vi "Chain2.vi"(7 "Name (\"\" to Use UUID)":string="CSM-Module") -> ()   [LabVIEW 2017, in "CSM-Testcase.lvlib"]
doc: "Creates a template for a CSM module without a user interface.\n\n> [!NOTE] CSM Name Rules\n> - The CSM module name must be unique to avoid entering the \"Critical Error\" state.\n> - If the input is \"\", a UUID will be used as the module name. This module will operate in independent mode and will not be listed in the module list.\n> - If the input ends with '#', the module will run in work mode. Modules with the same name will share the same message queue. External messages will be handled by the idle module.\n\n> [!NOTE] CSM Initialization State\n> - The default value is \"Macro: Initialize\", consistent with the JKISM state machine.\n> - This state is typically not modified and is provided to facilitate external programmatic changes to the initialization state.\n\n\n-- <b>Controls</b> --\n- <b>Name (\"\" to Use UUID)</b>: CSM Module Name\n- <b>Init State(\"Macro: Initialize\")</b>: Initialization State, default is \"Macro: Initialize\""
uses:
  CSM-Testcase.lvlib
  src/user.lib/_NEVSTOP/Communicable State Machine(CSM)/AdvanceAPI/CSM - Revert Arguments-Safe String.vi
  src/user.lib/_NEVSTOP/Communicable State Machine(CSM)/AdvanceAPI/CSM - Make String Arguments Safe.vi
  src/user.lib/_NEVSTOP/Communicable State Machine(CSM)/AdvanceAPI/CSM - Break Down Multiple States String.vi
  src/user.lib/_NEVSTOP/Communicable State Machine(CSM)/AdvanceAPI/CSM - Keywords.vi
  src/user.lib/_NEVSTOP/Communicable State Machine(CSM)/_Shared/Trim Single-line Text.vi
  src/user.lib/_NEVSTOP/Communicable State Machine(CSM)/_Polymophic/Build No-Reply Asynchronous Message with Arguments.vi
  src/user.lib/_NEVSTOP/Communicable State Machine(CSM)/_Polymophic/Build Asynchronous Message with Arguments.vi
  src/user.lib/_NEVSTOP/Communicable State Machine(CSM)/_Polymophic/Build Register Message.vi
  src/user.lib/_NEVSTOP/Communicable State Machine(CSM)/_Polymophic/Build Interrupt Broadcast Message.vi
  src/user.lib/_NEVSTOP/Communicable State Machine(CSM)/Communicable State Machine.lvlib
  src/user.lib/_NEVSTOP/Communicable State Machine(CSM)/addons/Loop-Support/CSM Loop Support.lvlib
panel:
  out "Error Occurred":errorcluster
  out "State History":string
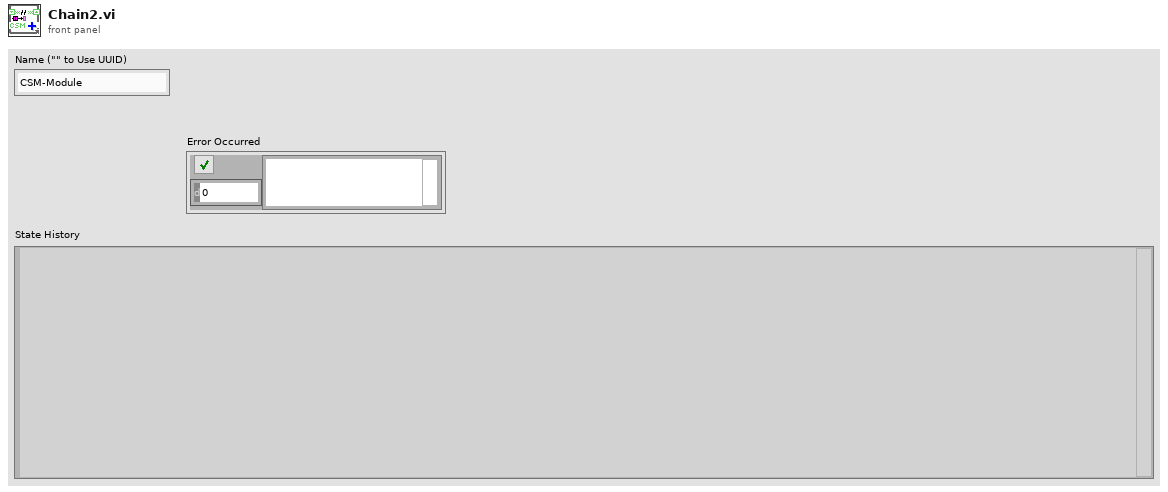
[diagram p1: front panel]
types:
  T1 = cluster{"Arguments":string, "Response":string, "error":errorcluster}
  T2 = enum32{"Invalid", "Standard", "Closed", "Hidden", "Minimized", "Maximized"}
  T3 = enum32{"invalid app kind", "Development System", "Run Time System", "Student Edition", "Embedded LabVIEW", "Evaluation", "Custom"}
  T4 = typedef "Communicable State Machine.lvlib/_CSM_Response Source Message.ctl" = cluster{"‘State":string, "’Arguments":string, "’Error":errorcluster}
  T5 = cluster{"Current VI Reference":refnum<vi>, "Close Panel on Exit?":bool}
  T6 = cluster{"Core":cluster{"Current VI Reference":refnum<vi>, "Close Panel on Exit?":bool}, "Your Boolean data":bool, "Your string data":string, "Counter":u32, "CSM Loop Counter":i32}
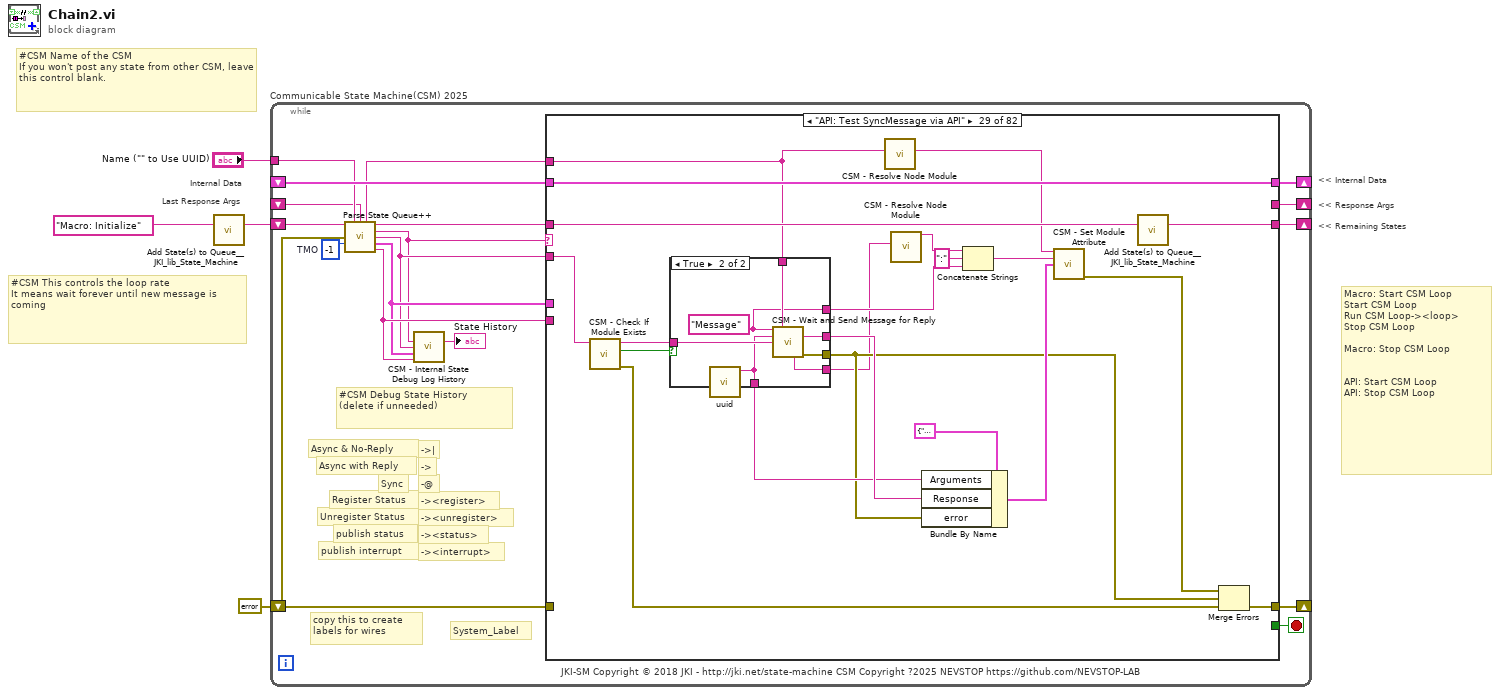
[diagram p0: block diagram]
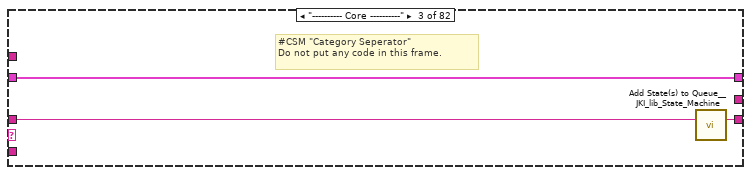
[diagram p4: hidden frame]
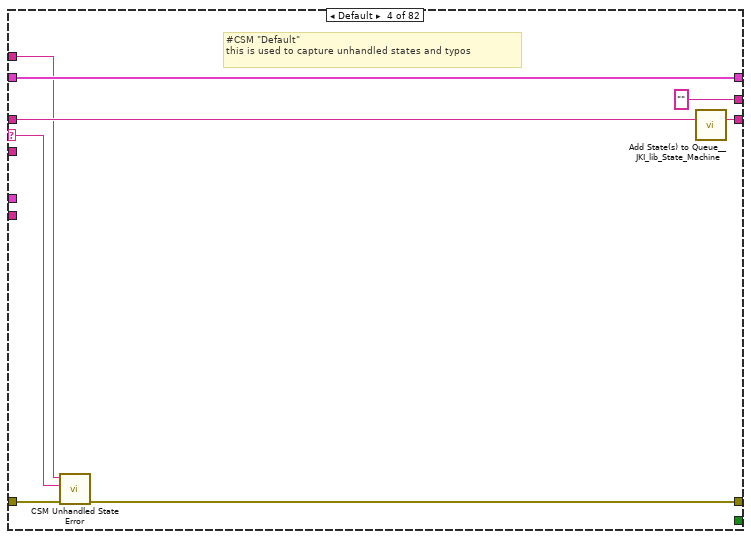
[diagram p5: hidden frame]
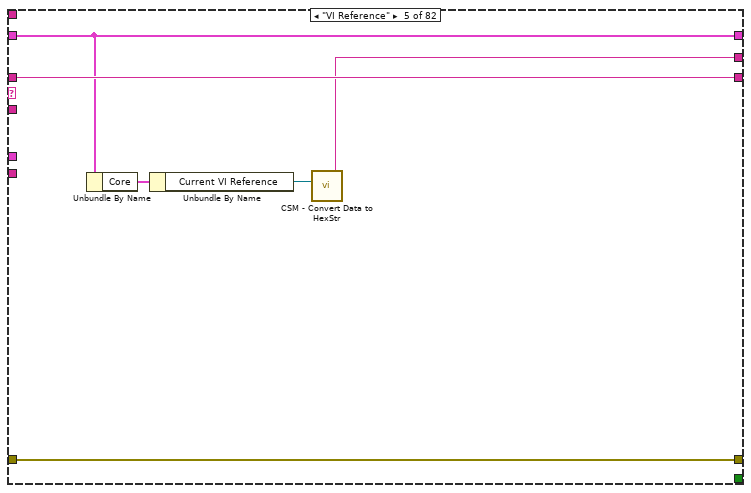
[diagram p6: hidden frame]
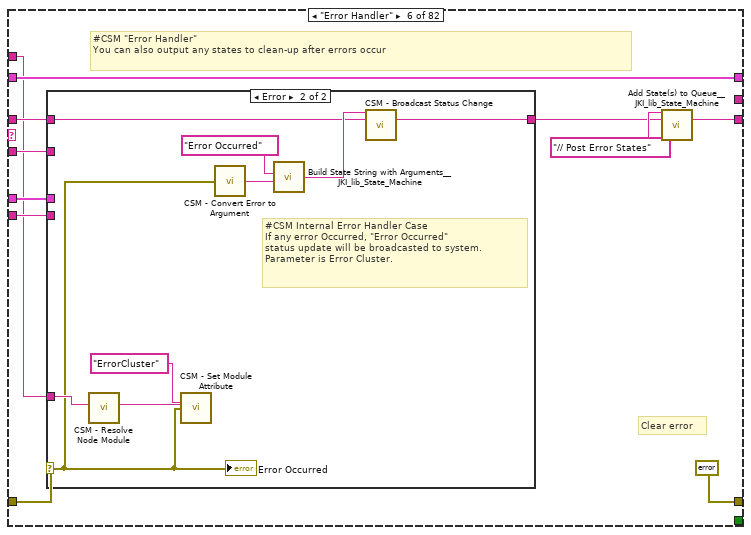
[diagram p7: hidden frame]
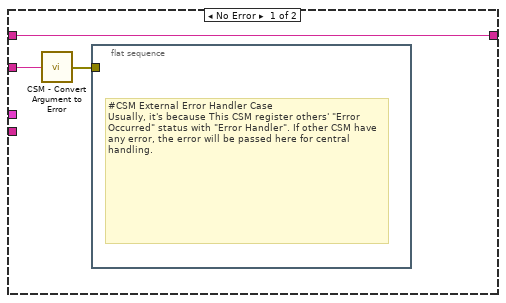
[diagram p8: hidden frame]
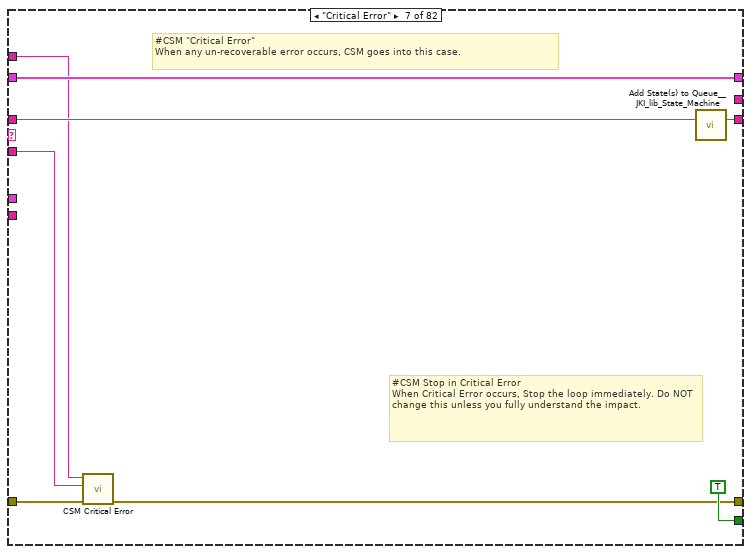
[diagram p9: hidden frame]
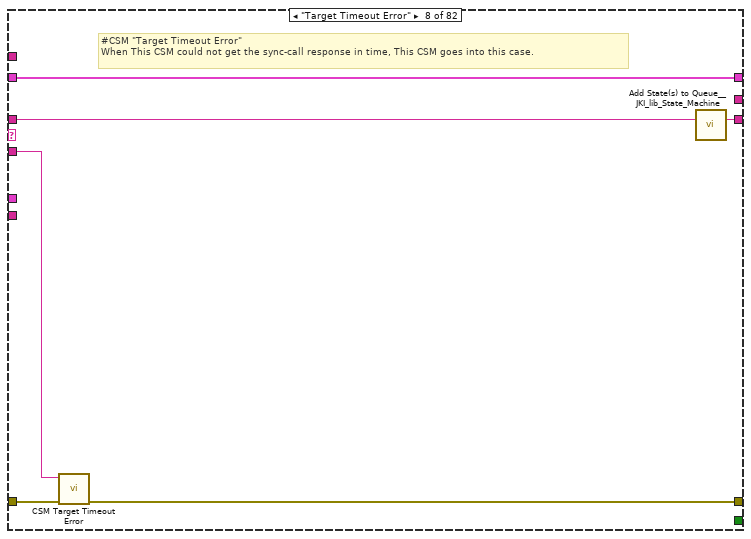
[diagram p10: hidden frame]
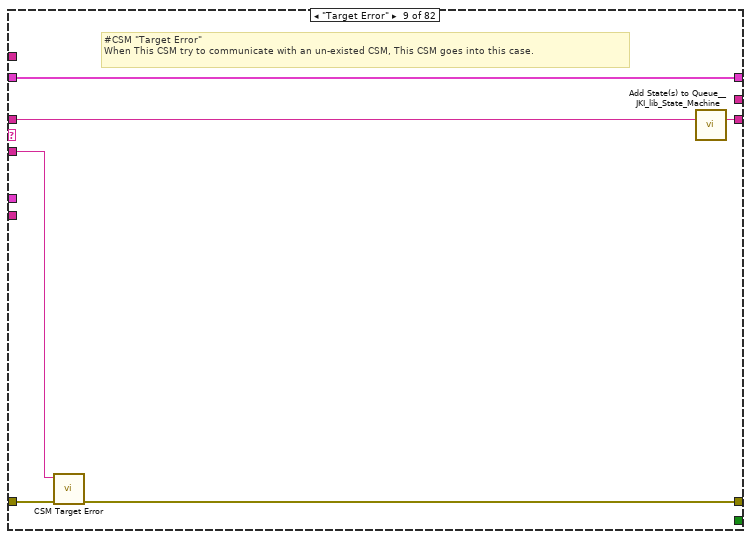
[diagram p11: hidden frame]
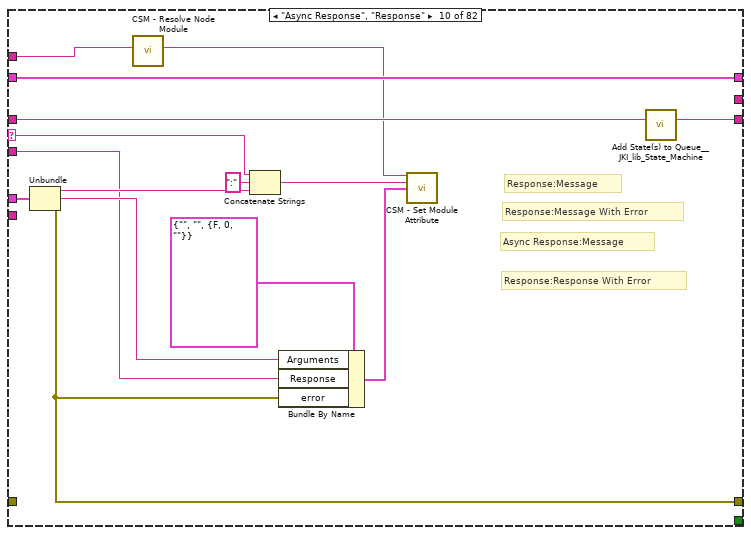
[diagram p12: hidden frame]
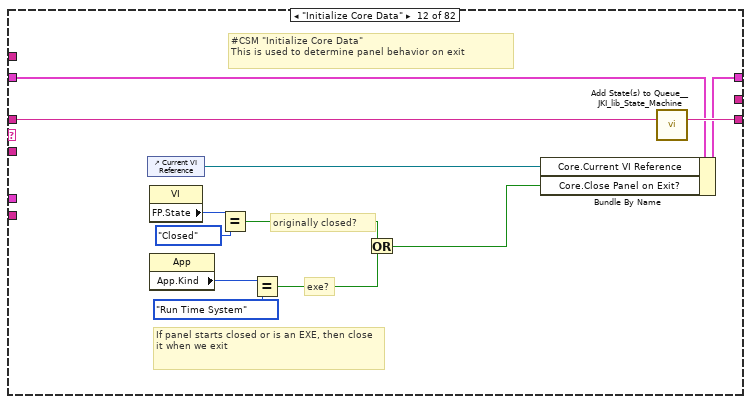
[diagram p14: hidden frame]
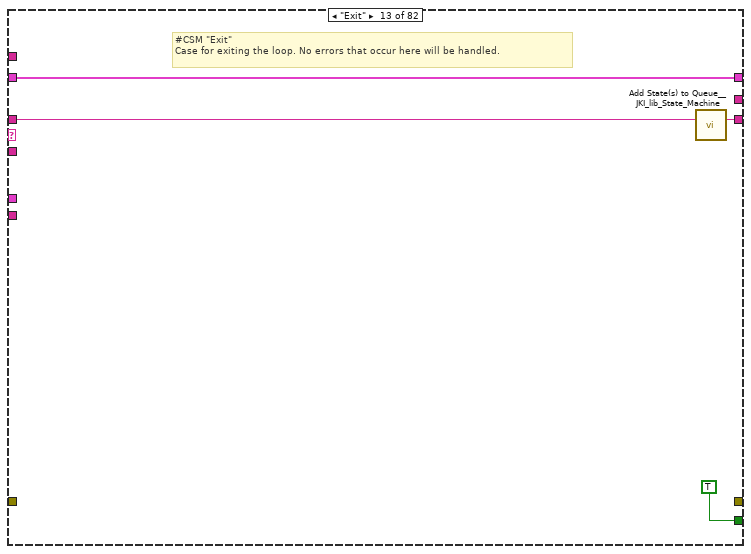
[diagram p15: hidden frame]
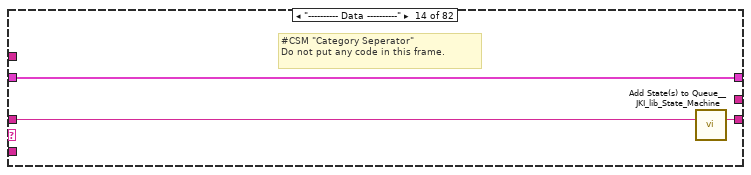
[diagram p16: hidden frame]
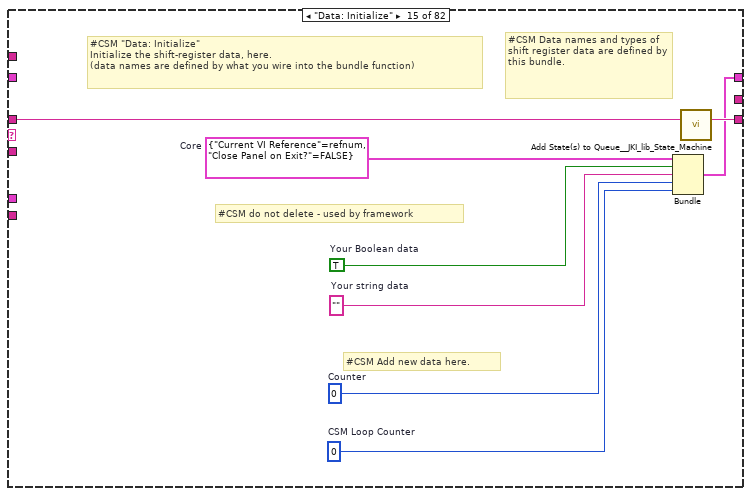
[diagram p17: hidden frame]
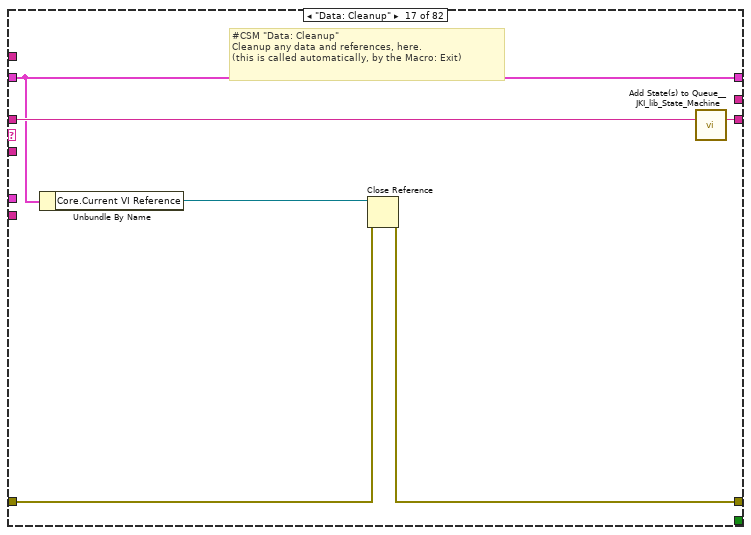
[diagram p19: hidden frame]
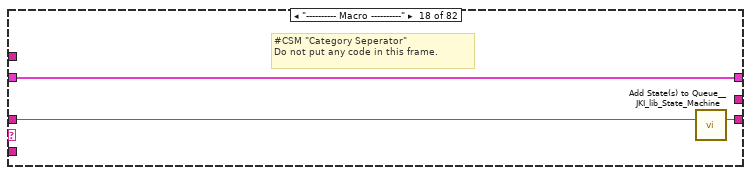
[diagram p20: hidden frame]
diagram:
  # "Macro: Start CSM Loop\nStart CSM Loop\nRun CSM Loop-><loop>\nStop CSM Loop\n\nMacro: Stop CSM Loop\n\n\nAPI: Start CSM Loop\nAPI: Stop CSM Loop"
  # "Last Response Args"
  # "Internal Data"
  # "#CSM Name of the CSM\nIf you won't post any state from other CSM, leave this control blank."
  # "#CSM This controls the loop rate\nIt means wait forever until new message is coming"
  # "<< Internal Data"
  # "<< Response Args"
  # "<< Remaining States"
  n1 = call <vilib>:"Add State(s) to Queue__JKI_lib_State_Machine.vi"("State(s) in (\"\")"="Macro: Initialize" ("Init State(\"Macro: Initialize\")")) -> ("States Out"=w4:string)  [unwired: 14 in]
  n2 = while "Communicable State Machine(CSM) 2025" {
    shift-right: [w17] -> _
    shift-left: _ -> [w16]
    shift-right: [w20] -> _
    shift-left: errorcluster {"status"=FALSE, "code"=0, "source"=""} ("error out") -> [w6]
    shift-right: [w19] -> _
    shift-left: w4 -> [w21]
    tunnel: "Name (\"\" to Use UUID)" -> [w13]
    shift-right: [w14] -> _
    shift-left: _ -> [w8]
    stop <- w18 stop-if-true
    w15 = -1  # TMO
    # "#CSM Debug State History\n(delete if unneeded)"
    # "-><interrupt>"
    # "-><status>"
    # "-><unregister>"
    # "-><register>"
    # "-@"
    # "->"
    # "->|"
    # "publish interrupt"
    # "publish status"
    # "Unregister Status"
    # "Register Status"
    # "Sync"
    # "Async with Reply"
    # "Async & No-Reply"
    # "JKI-SM Copyright © 2018 JKI - http://jki.net/state-machine CSM Copyright ?2025 NEVSTOP https://github.com/NEVSTOP-LAB"
    # "copy this to create labels for wires"
    # "System_Label"
    n3 = call "Parse State Queue++.vi"("State Queue"=w21, "Name (\"\" to Use UUID)"=w13, "Response Arguments"=w8, "Previous Error"=w6, "Dequeue (1 ms)"=w15) -> ("Name Used"=w7:string, "Remaining States"=w22:string, "Current State"=w9:string, "Arguments"=w10:string, "Additional Information"=w11:T4, "Source CSM"=w12:string)  [unwired: 5 in]
    n4 = call "CSM - Internal State Debug Log History.vi"("State"=w9, "Arguments (\"\")"=w10, ">> Response Source Message >>"=w11, "Source (\"\")"=w12) -> ("Debug Log"=→"State History":string)  [unwired: 11 in]
    n5 = case shown="\"API: Test SyncMessage via API\"" w9 {
      selector: w9 -> [_ _ _ w33 _ _ _ _ _ w97 _ _ _ _ _ _ _ _ _ _ _ _ _ _ _ _ _ _ _ _ _ _ _ _ _ _ _ _ _ _ _ _ _ _ _ _ _ _ _ _ _ _ _ _ _ _ _ _ _ w549 w559 _ w573 _ _ _ _ _ _ _ _ _ _ w639 _ _ _ w663 w674 w681 w696 _]
      tunnel: w22 -> [w23 w26 w29 w37 w42 w48 w74 w80 w86 w101 w103 w115 w119 w122 w130 w132 w138 w141 w145 w151 w155 w160 w174 w194 w223 w227 w231 w243 w268 w296 w311 w323 w335 w349 w372 w383 w396 w403 w410 w417 w424 w431 w438 w445 w452 w459 w466 w473 w484 w492 w501 w510 w519 w522 w526 w533 w538 w541 w545 w557 w567 w572 w578 w585 w588 w600 w606 w612 w616 w621 w625 w629 w633 w642 w646 w654 w660 w667 w676 w685 w700 w710]
      tunnel: w10 -> [_ _ _ _ _ w47 w70 w77 w83 w91 _ _ _ _ _ _ _ _ _ _ _ _ w161 w181 w206 _ w234 w246 w271 w299 w314 w326 w338 w352 w368 w386 w393 w400 w407 w414 w421 w428 w435 w442 w449 w456 w463 w470 w477 _ w494 w502 w511 _ _ w531 _ _ _ _ _ w569 _ w581 w590 _ w602 w608 w614 w619 w624 w628 w632 w638 w645 w652 w658 w664 w675 w680 w691 _]
      tunnel: w16 -> [w24 w25 w27 w35 w41 w53 w72 w78 w84 w99 w102 w109 w117 w120 _ w131 w133 w139 w143 w149 w156 w158 w176 w196 w225 w226 w235 w247 w272 w300 w315 w327 w339 w353 w375 w387 w398 w405 w412 w419 w426 w433 w440 w447 w454 w461 w468 w475 w482 w490 w499 w508 w517 w523 w528 w532 w536 w539 w544 w555 w565 w570 w579 w586 w592 w601 w607 w613 w618 w623 w626 w630 w634 w643 w647 w653 w659 w668 w677 w686 w693 w708]
      tunnel: [_ _ _ w30 w43 errorcluster {"status"=FALSE, "code"=0, "source"=""} ("error out") w67 w75 w81 w90 _ _ _ _ _ _ w134 _ _ _ _ _ _ _ _ _ w228 w240 w265 w293 w308 w320 w332 w345 w369 w380 w397 w404 w411 w418 w425 w432 w439 w446 w453 w460 w467 w474 _ _ _ w506 w515 w524 w529 _ _ _ w546 w547 w562 _ _ _ _ _ _ _ w617 w622 w627 w631 w635 w637 w648 w649 w655 w662 w671 w682 w697 _] -> w20
      tunnel: w6 -> [_ _ _ w31 w43 w51 w68 w76 w82 _ _ _ _ _ _ _ w135 _ _ _ _ _ _ _ _ _ _ _ _ _ _ _ _ _ _ _ w397 w404 w411 w418 w425 w432 w439 w446 w453 w460 w467 w474 _ _ _ _ _ w524 w529 _ _ _ w546 _ _ _ _ _ _ _ _ _ w617 w622 w627 w631 w635 w644 w648 w650 w656 w669 w678 w687 w701 _]
      tunnel: [w23 w26 w28 w36 w42 w49 w73 w79 w85 w100 w103 w114 w118 w121 w129 w132 w137 w140 w144 w150 w152 w159 w175 w195 w224 w227 w232 w244 w269 w297 w312 w324 w336 w350 w373 w384 w395 w402 w409 w416 w423 w430 w437 w444 w451 w458 w465 w472 w483 w491 w500 w509 w518 w521 w525 w533 w537 w540 w545 w558 w568 w571 w580 w582 w587 w598 w603 w609 w615 w620 w625 w629 w633 w642 w646 w654 w660 w667 w676 w685 w700 w709] -> w19
      tunnel: [_ _ _ _ _ _ TRUE _ _ _ _ _ TRUE _ _ _ _ _ _ _ _ _ _ _ _ _ _ _ _ _ _ _ _ _ _ _ _ _ _ _ _ _ _ _ _ _ _ _ _ _ _ _ _ _ _ _ _ _ _ _ _ _ _ _ _ _ _ _ _ _ _ _ _ _ _ _ _ _ _ _ _ _] -> w18
      tunnel: [w24 w25 w27 w35 w41 w53 w72 w78 w84 w99 w102 w113 w117 w120 w128 w131 w133 w139 w143 w149 w156 w158 w176 w196 w225 w226 w235 w247 w272 w300 w315 w327 w339 w353 w375 w387 w398 w405 w412 w419 w426 w433 w440 w447 w454 w461 w468 w475 w482 w490 w499 w508 w517 w523 w528 w532 w536 w539 w543 w553 w564 w570 w579 w586 w592 w601 w607 w613 w618 w623 w626 w630 w634 w643 w647 w653 w659 w668 w677 w686 w692 w706] -> w17
      tunnel: w12 -> [_ _ _ _ _ w46 _ _ _ _ _ _ _ _ _ _ _ _ _ _ _ _ _ _ _ _ _ _ _ _ _ _ _ _ _ _ _ _ _ _ _ _ _ _ _ _ _ _ _ _ _ _ _ _ _ _ _ _ _ _ _ _ _ _ _ _ _ _ _ _ _ _ _ _ _ _ _ _ _ _ _ _]
      tunnel: w11 -> [_ _ _ _ _ w45 _ _ _ w98 _ _ _ _ _ _ _ _ _ _ _ _ _ _ _ _ _ _ _ _ _ _ _ _ _ _ _ _ _ _ _ _ _ _ _ _ _ _ _ _ _ _ _ _ _ _ _ _ _ _ _ _ _ _ _ _ _ _ _ _ _ _ _ _ _ _ _ _ _ _ _ _]
      tunnel: [_ _ _ "" w38 _ _ _ _ _ _ _ _ _ _ _ _ _ _ _ _ _ _ _ _ _ _ _ _ _ _ _ _ _ _ _ _ _ _ _ _ _ _ _ _ _ _ _ _ _ _ _ _ _ _ w530 _ _ _ _ _ w569 w574 _ _ _ _ _ w614 w619 w624 w628 w632 w638 w645 w652 w658 _ w675 w680 _ _] -> w14
      tunnel: w7 -> [_ _ _ w32 _ w44 w69 _ _ w88 _ _ _ _ _ _ _ _ _ _ _ _ _ _ _ _ _ _ w256 w284 _ _ _ w346 _ _ _ _ _ _ _ _ _ _ _ _ _ _ w480 w488 w497 w507 w516 _ _ _ _ _ _ w551 w561 _ w575 _ _ w595 _ _ _ _ _ _ _ w641 _ _ _ w666 w673 w684 w699 _]
      frame "", "Idle" {
        # "#CSM \"Idle/Event Handler\"\nexecutes when the state queue is empty"
      }
      frame "CSM Documentation" {
        # "#CSM State Syntax\n\n// Comment line, all text to the right of “//” will be ignored\n// Local Message Example\nDoSth: DoA >> Arguments\n\n// Sync Call Example\nAPI: xxxx >> Arguments -@ TargetModule\n\n// Async Call Example\nAPI: xxxx >> Arguments -> TargetModule\n\n// Async Call without Reply Example\nAPI: xxxx >> Arguments ->| TargetModule\n\n// Broadcast normal status:\nStatus >> StatusArguments  -><status>\n\n// Broadcast Interrupt status:\nInterrupt >> StatusArguments  -><interrupt>\n\n// Register Source Module's status to Handler Module\nStatus@Source Module >> Handler Module@Handler Module -><register>\n\n// Unegister Source Module's status\nStatus@Source Module >> Handler Module -><unregister>"
        # "#CSM README FIRST\n\nCommunicable State Machine(CSM) is a LabVIEW application framework that builds upon JKI State Machine(JKISM). It follows the pattern of JKISM and extends the keywords to describe message communication between modules, including concepts such as Sync-Message, Async-Message, Subscription/Unsubscription of status - essential elements for creating reusable code modules. For more information, please visit the CSM wiki: https://nevstop-lab.github.io/CSM-Wiki/\n\nFor instructions on JKI State Machine, visit: \n    http://jki.net/state-machine/\nFor information about CSM, visit: \n    https://github.com/NEVSTOP-LAB"
        # "#CSM \"Documentation\"\nCase for holding CSM Documenation"
      }
      frame "---------- Core ----------" {
        # "#CSM \"Category Seperator\"\nDo not put any code in this frame."
        n6 = call <vilib>:"Add State(s) to Queue__JKI_lib_State_Machine.vi"("State(s) in (\"\")"=w29) -> ("States Out"=w28:string)  [unwired: 14 in]
      }
      frame Default {
        # "#CSM \"Default\"\nthis is used to capture unhandled states and typos"
        n7 = call "CSM Unhandled State Error.vi"("error in (no error)"=w31, "Undefined State"=w33, "CSM Name"=w32) -> ("error out"=w30:errorcluster)  [unwired: 8 in]
        n8 = call <vilib>:"Add State(s) to Queue__JKI_lib_State_Machine.vi"("State(s) in (\"\")"=w37) -> ("States Out"=w36:string)  [unwired: 14 in]
      }
      frame "VI Reference" {
        n9 = Unbundle By Name(w41) -> ("Core"=w40:T5)
        n10 = Unbundle By Name(w40) -> ("Current VI Reference"=w39:refnum<vi>)
        n11 = call "CSM - Convert Data to HexStr.vi"("Variant"=w39) -> ("HEX String (0-9,A-F)"=w38:string)  [unwired: 8 in]
      }
      frame "Error Handler" {
        # "#CSM \"Error Handler\"\nYou can also output any states to clean-up after errors occur"
        # "Clear error"
        n12 = case shown="Error" w51 {
          selector: w51 -> [_ w59]
          tunnel: [w57 w63] -> w50
          tunnel: w48 -> [w57 w62]
          tunnel: w47 -> [w56 _]
          tunnel: w46 -> [_ _]
          tunnel: w45 -> [_ _]
          tunnel: w44 -> [_ w61]
          frame No Error {
            n13 = call "CSM - Convert Argument to Error.vi"("Argument"=w56) -> ("Error"=w55:errorcluster)  [unwired: 4 in]
            n14 = flat-sequence {
              tunnel: w55 -> [_]
              frame #0 {
                # "#CSM External Error Handler Case\nUsually, it's because This CSM register others' \"Error Occurred\" status with \"Error Handler\". If other CSM have any error, the error will be passed here for central handling."
              }
            }
          }
          frame Error {
            # "#CSM Internal Error Handler Case \nIf any error Occurred, \"Error Occurred\" \nstatus update will be broadcasted to system.\nParameter is Error Cluster."
            n15 = call "CSM - Resolve Node Module.vi"("Node Name"=w61) -> ("CSM Module Name"=w60:string)  [unwired: 10 in]
            n16 = call "CSM - Set Module Attribute.vi"("CSM Name"=w60, "Attribute"="ErrorCluster", "Value"=w59) -> ()  [unwired: 9 in, 4 out]
            n17 = call "CSM - Convert Error to Argument.vi"("Error"=w59) -> ("Argument"=w65:string)  [unwired: 4 in]
            n18 = call <vilib>:"Build State String with Arguments__JKI_lib_State_Machine.vi"("Arguments (\"\")"=w65, "State"="Error Occurred" ("Status with Arguments")) -> ("State with Arguments"=w64:string)  [unwired: 4 in]
            n19 = call "CSM - Broadcast Status Change.vi"("Status With Arguments"=w64, "State Queue"=w62) -> ("Remaining States"=w63:string)  [unwired: 13 in]
            "Error Occurred" <- w59
          }
        }
        n20 = call <vilib>:"Add State(s) to Queue__JKI_lib_State_Machine.vi"("State(s) in Front (\"\")"="// Post Error States", "State(s) in (\"\")"=w50) -> ("States Out"=w49:string)  [unwired: 13 in]
      }
      frame "Critical Error" {
        # "#CSM \"Critical Error\"\nWhen any un-recoverable error occurs, CSM goes into this case."
        # "#CSM Stop in Critical Error\nWhen Critical Error occurs, Stop the loop immediately. Do NOT change this unless you fully understand the impact."
        n21 = call "CSM Critical Error.vi"("error in (no error)"=w68, "Arugments (As Reason)"=w70, "CSM Name"=w69) -> ("error out"=w67:errorcluster)  [unwired: 8 in]
        n22 = call <vilib>:"Add State(s) to Queue__JKI_lib_State_Machine.vi"("State(s) in (\"\")"=w74) -> ("States Out"=w73:string)  [unwired: 14 in]
      }
      frame "Target Timeout Error" {
        # "#CSM \"Target Timeout Error\"\nWhen This CSM could not get the sync-call response in time, This CSM goes into this case."
        n23 = call "CSM Target Timeout Error.vi"("error in (no error)"=w76, "Arguments (As CSM Name)"=w77) -> ("error out"=w75:errorcluster)  [unwired: 9 in]
        n24 = call <vilib>:"Add State(s) to Queue__JKI_lib_State_Machine.vi"("State(s) in (\"\")"=w80) -> ("States Out"=w79:string)  [unwired: 14 in]
      }
      frame "Target Error" {
        # "#CSM \"Target Error\"\nWhen This CSM try to communicate with an un-existed CSM, This CSM goes into this case."
        n25 = call "CSM Target Error.vi"("error in (no error)"=w82, "Arguments (As CSM Name)"=w83) -> ("error out"=w81:errorcluster)  [unwired: 9 in]
        n26 = call <vilib>:"Add State(s) to Queue__JKI_lib_State_Machine.vi"("State(s) in (\"\")"=w86) -> ("States Out"=w85:string)  [unwired: 14 in]
      }
      frame "Async Response", "Response" {
        # "Response:Response With Error"
        # "Response:Message With Error"
        # "Async Response:Message"
        # "Response:Message"
        n27 = Unbundle(w98) -> ("‘State"=w96:string, "’Arguments"=w92:string, "’Error"=w90:errorcluster)
        n28 = call "CSM - Resolve Node Module.vi"("Node Name"=w88) -> ("CSM Module Name"=w87:string)  [unwired: 10 in]
        n29 = Concatenate Strings(w97, ":" ("string"), w96) -> (w94:string)
        n30 = Bundle By Name(cluster=T1 {"Arguments"="", "Response"="", "error"={"status"=FALSE, "code"=0, "source"=""}}, "Arguments"=w92, "Response"=w91, "error"=w90) -> (w89:T1)
        n31 = call "CSM - Set Module Attribute.vi"("CSM Name"=w87, "Attribute"=w94, "Value"=w89) -> ()  [unwired: 9 in, 4 out]
        n32 = call <vilib>:"Add State(s) to Queue__JKI_lib_State_Machine.vi"("State(s) in (\"\")"=w101) -> ("States Out"=w100:string)  [unwired: 14 in]
      }
      frame "Async Message Posted" {
        # "#CSM \"Async Message Posted\"\nAfter Async Message is posted (-> or ->| ), CSM goes to this state for post-action.\nYou can use Argument - State to tell which Async Message is called."
      }
      frame "Initialize Core Data" {
        # "#CSM \"Initialize Core Data\"\nThis is used to determine panel behavior on exit"
        # "originally closed?"
        # "exe?"
        # "If panel starts closed or is an EXE, then close it when we exit"
        n33 = control-ref of="Current VI Reference"() -> (w107:refnum<vi>)
        n34 = property class="VI"() -> ("FP.State"=w106:T2)  [unwired: 2 in, 2 out]
        n35 = property class="App"() -> ("App.Kind"=w112:T3)  [unwired: 2 in, 2 out]
        n36 = Equal?(x=w106, y=T2."Closed" ("Front Panel Window:State")) -> (x = y?=w104:bool)
        n37 = Equal?(x=w112, y=T3."Run Time System" ("Application:Kind")) -> (x = y?=w110:bool)
        n38 = Or(x=w104, y=w110) -> (x .or. y?=w108:bool)
        n39 = Bundle By Name(cluster=w109, "Core.Current VI Reference"=w107, "Core.Close Panel on Exit?"=w108) -> (w113:T6)
        n40 = call <vilib>:"Add State(s) to Queue__JKI_lib_State_Machine.vi"("State(s) in (\"\")"=w115) -> ("States Out"=w114:string)  [unwired: 14 in]
      }
      frame "Exit" {
        # "#CSM \"Exit\"\nCase for exiting the loop. No errors that occur here will be handled."
        n41 = call <vilib>:"Add State(s) to Queue__JKI_lib_State_Machine.vi"("State(s) in (\"\")"=w119) -> ("States Out"=w118:string)  [unwired: 14 in]
      }
      frame "---------- Data ----------" {
        # "#CSM \"Category Seperator\"\nDo not put any code in this frame."
        n42 = call <vilib>:"Add State(s) to Queue__JKI_lib_State_Machine.vi"("State(s) in (\"\")"=w122) -> ("States Out"=w121:string)  [unwired: 14 in]
      }
      frame "Data: Initialize" {
        w123 = 0  # CSM Loop Counter
        w124 = u32 0  # Counter
        w125 = T5 {"Current VI Reference"=refnum, "Close Panel on Exit?"=FALSE}  # Core
        w127 = TRUE  # Your Boolean data
        w126 = ""  # Your string data
        # "#CSM \"Data: Initialize\"\nInitialize the shift-register data, here.\n(data names are defined by what you wire into the bundle function)"
        # "#CSM do not delete - used by framework"
        # "#CSM Add new data here."
        # "#CSM Data names and types of shift register data are defined by this bundle."
        n43 = Bundle("Core"=w125, "Your Boolean data"=w127, "Your string data"=w126, "Counter"=w124, "CSM Loop Counter"=w123) -> (w128:T6)  [unwired: 1 in]
        n44 = call <vilib>:"Add State(s) to Queue__JKI_lib_State_Machine.vi"("State(s) in (\"\")"=w130) -> ("States Out"=w129:string)  [unwired: 14 in]
      }
      frame "Data: Update Indicators" {
      }
      frame "Data: Cleanup" {
        # "#CSM \"Data: Cleanup\"\nCleanup any data and references, here.\n(this is called automatically, by the Macro: Exit)"
        n45 = Unbundle By Name(w133) -> ("Core.Current VI Reference"=w136:refnum<vi>)
        n46 = Close Reference(reference=w136, error in (no error)=w135) -> (error out=w134:errorcluster)
        n47 = call <vilib>:"Add State(s) to Queue__JKI_lib_State_Machine.vi"("State(s) in (\"\")"=w138) -> ("States Out"=w137:string)  [unwired: 14 in]
      }
      frame "---------- Macro ----------" {
        # "#CSM \"Category Seperator\"\nDo not put any code in this frame."
        n48 = call <vilib>:"Add State(s) to Queue__JKI_lib_State_Machine.vi"("State(s) in (\"\")"=w141) -> ("States Out"=w140:string)  [unwired: 14 in]
      }
      frame "Macro: Initialize" {
        # "#CSM \"Macro: Initialize\"\nInitialization Macro (This is called once, when the VI starts)"
        n49 = call <vilib>:"Add State(s) to Queue__JKI_lib_State_Machine.vi"("State(s) in Front (\"\")"="Data: Initialize\nInitialize Core Data\nData: Update Indicators", "State(s) in (\"\")"=w145) -> ("States Out"=w144:string)  [unwired: 13 in]
      }
      frame "Macro: Exit" {
        # "#CSM \"Macro: Exit\"\nExit Macro (This is called once, when the VI exits)"
        n50 = call <vilib>:"Add State(s) to Queue__JKI_lib_State_Machine.vi"("State(s) in Front (\"\")"="//Exit Sub-Modules ", "State(s) at Back (\"\")"="Data: Cleanup\nExit") -> ("States Out"=w147:string)  [unwired: 13 in]
        n51 = call <vilib>:"Add State(s) to Queue__JKI_lib_State_Machine.vi"("State(s) in Front (\"\")"=w147, "State(s) in (\"\")"=w151) -> ("States Out"=w150:string)  [unwired: 13 in]
      }
      frame "Macro: Start CSM Loop" {
        n52 = call "CSMLS - Define Loop State(s).vi"("Loop States"="Start CSM Loop\nRun CSM Loop-><loop>\nStop CSM Loop", "States Queue"=w155, "Add to Front? (F)"=FALSE) -> ("Remaining States"=w152:string)  [unwired: 12 in]
      }
      frame "Macro: Stop CSM Loop" {
        n53 = call <vilib>:"Add State(s) to Queue__JKI_lib_State_Machine.vi"("State(s) in Front (\"\")"="Stop CSM Loop", "State(s) in (\"\")"=w160) -> ("States Out"=w159:string)  [unwired: 13 in]
      }
      frame "Macro: Test MacroWithSubMessages" {
        w162 = "SubMessage2" ("State With Arguments")
        w164 = "SubMessage1" ("State With Arguments")
        n54 = call "uuid.vi"() -> ("UUID"=w163:string)  [unwired: 11 in]
        n55 = call "uuid.vi"() -> ("UUID"=w165:string)  [unwired: 11 in]
        n56 = Concatenate Strings(w164, w165) -> (w166:string)
        n57 = Concatenate Strings(w162, w163) -> (w167:string)
        n58 = call <vilib>:"Build State String with Arguments__JKI_lib_State_Machine.vi"("Arguments (\"\")"=w161, "State"="SubMessage3" ("State With Arguments")) -> ("State with Arguments"=w169:string)  [unwired: 4 in]
        n59 = call <vilib>:"Build State String with Arguments__JKI_lib_State_Machine.vi"("Arguments (\"\")"=w166, "State"=w164) -> ("State with Arguments"=w171:string)  [unwired: 4 in]
        n60 = call <vilib>:"Build State String with Arguments__JKI_lib_State_Machine.vi"("Arguments (\"\")"=w167, "State"=w162) -> ("State with Arguments"=w170:string)  [unwired: 4 in]
        n61 = Build Array(w171, w170, w169) -> (w168:string[])
        n62 = call "CSM - Compact Multiple States.vi"("Multiple States"=w168) -> ("States"=w173:string)  [unwired: 9 in]
        n63 = call <vilib>:"Add State(s) to Queue__JKI_lib_State_Machine.vi"("State(s) in Front (\"\")"=w173, "State(s) in (\"\")"=w174) -> ("States Out"=w175:string)  [unwired: 13 in]
      }
      frame "Macro: Test MacroWithSubAndPostMessages" {
        w180 = "PostMessage1" ("State With Arguments")
        w182 = "SubMessage2" ("State With Arguments")
        w184 = "SubMessage1" ("State With Arguments")
        n64 = call "uuid.vi"() -> ("UUID"=w183:string)  [unwired: 11 in]
        n65 = call "uuid.vi"() -> ("UUID"=w179:string)  [unwired: 11 in]
        n66 = call "uuid.vi"() -> ("UUID"=w185:string)  [unwired: 11 in]
        n67 = Concatenate Strings(w180, w179) -> (w178:string)
        n68 = Concatenate Strings(w184, w185) -> (w186:string)
        n69 = Concatenate Strings(w182, w183) -> (w187:string)
        n70 = call <vilib>:"Build State String with Arguments__JKI_lib_State_Machine.vi"("Arguments (\"\")"=w181, "State"="SubMessage3" ("State With Arguments")) -> ("State with Arguments"=w189:string)  [unwired: 4 in]
        n71 = call <vilib>:"Build State String with Arguments__JKI_lib_State_Machine.vi"("Arguments (\"\")"=w178, "State"=w180) -> ("State with Arguments"=w177:string)  [unwired: 4 in]
        n72 = call <vilib>:"Build State String with Arguments__JKI_lib_State_Machine.vi"("Arguments (\"\")"=w186, "State"=w184) -> ("State with Arguments"=w191:string)  [unwired: 4 in]
        n73 = call <vilib>:"Build State String with Arguments__JKI_lib_State_Machine.vi"("Arguments (\"\")"=w187, "State"=w182) -> ("State with Arguments"=w190:string)  [unwired: 4 in]
        n74 = Build Array(w191, w190, w189) -> (w188:string[])
        n75 = call "CSM - Compact Multiple States.vi"("Multiple States"=w188) -> ("States"=w193:string)  [unwired: 9 in]
        n76 = call <vilib>:"Add State(s) to Queue__JKI_lib_State_Machine.vi"("State(s) in Front (\"\")"=w193, "State(s) in (\"\")"=w194, "State(s) at Back (\"\")"=w177) -> ("States Out"=w195:string)  [unwired: 12 in]
      }
      frame "Macro: TestMacroWithNonLocalSubMessages" {
        w210 = "PostMessage1" ("State With Arguments")
        w211 = "SubMessage2" ("State With Arguments")
        w213 = "SubMessage1" ("State With Arguments")
        n77 = Match Pattern(string=w206, regular expression="+") -> (before substring=w198:string, after substring=w197:string)  [unwired: 1 in, 2 out]
        n78 = call "uuid.vi"() -> ("UUID"=w209:string)  [unwired: 11 in]
        n79 = call "uuid.vi"() -> ("UUID"=w212:string)  [unwired: 11 in]
        n80 = call "uuid.vi"() -> ("UUID"=w214:string)  [unwired: 11 in]
        n81 = Concatenate Strings(w210, w209) -> (w208:string)
        n82 = Concatenate Strings(w213, w214) -> (w215:string)
        n83 = Concatenate Strings(w211, w212) -> (w216:string)
        n84 = call <vilib>:"Build State String with Arguments__JKI_lib_State_Machine.vi"("Arguments (\"\")"=w208, "State"=w210) -> ("State with Arguments"=w207:string)  [unwired: 4 in]
        n85 = call-poly "Build Message with Arguments++.vi"("State With Arguments"="SubMessage1", "Target Module (\"\")"=w197) -> ("CSM Message String"=w202:string)  [unwired: 13 in]
        n86 = call-poly "Build Message with Arguments++.vi"("State With Arguments"="SubMessage2", "Target Module (\"\")"=w197) -> ("CSM Message String"=w201:string)  [unwired: 13 in]
        n87 = call <vilib>:"Build State String with Arguments__JKI_lib_State_Machine.vi"("Arguments (\"\")"=w198, "State"="SubMessage3" ("State With Arguments")) -> ("State with Arguments"=w218:string)  [unwired: 4 in]
        n88 = call-poly "Build Message with Arguments++.vi"("State With Arguments"="Message", "Target Module (\"\")"=w197) -> ("CSM Message String"=w203:string)  [unwired: 13 in]
        n89 = call <vilib>:"Build State String with Arguments__JKI_lib_State_Machine.vi"("Arguments (\"\")"=w215, "State"=w213) -> ("State with Arguments"=w220:string)  [unwired: 4 in]
        n90 = call <vilib>:"Build State String with Arguments__JKI_lib_State_Machine.vi"("Arguments (\"\")"=w216, "State"=w211) -> ("State with Arguments"=w219:string)  [unwired: 4 in]
        n91 = Build Array(w220, w219, w218, w203, w202, w201) -> (w217:string[])
        n92 = call "CSM - Compact Multiple States.vi"("Multiple States"=w217) -> ("States"=w222:string)  [unwired: 9 in]
        n93 = call <vilib>:"Add State(s) to Queue__JKI_lib_State_Machine.vi"("State(s) in Front (\"\")"=w222, "State(s) in (\"\")"=w223, "State(s) at Back (\"\")"=w207) -> ("States Out"=w224:string)  [unwired: 12 in]
      }
      frame "---------- API ----------" {
        # "#CSM \"Category Seperator\"\nDo not put any code in this frame."
      }
      frame "API: Test SyncMessage" {
        n94 = call "CSM - Check If Module Exists.vi"("CSM Name"=w234) -> ("error out"=w228:errorcluster, "Exist?"=w229:bool, "CSM Name (Dup)"=w233:string)  [unwired: 8 in]
        n95 = case shown="True" w229 {
          tunnel: w233 -> [_ w237]
          tunnel: [_ w236] -> w230
          frame False {
          }
          frame True {
            n96 = call "uuid.vi"() -> ("UUID"=w238:string)  [unwired: 11 in]
            n97 = call-poly "Build Message with Arguments++.vi"("State With Arguments"="Message", "Arguments (\"\")"=w238, "Target Module (\"\")"=w237) -> ("CSM Message String"=w236:string)  [unwired: 12 in]
          }
        }
        n98 = call <vilib>:"Add State(s) to Queue__JKI_lib_State_Machine.vi"("State(s) in Front (\"\")"=w230, "State(s) in (\"\")"=w231) -> ("States Out"=w232:string)  [unwired: 13 in]
      }
      frame "API: Test SyncMessage With Error" {
        n99 = call "CSM - Check If Module Exists.vi"("CSM Name"=w246) -> ("error out"=w240:errorcluster, "Exist?"=w241:bool, "CSM Name (Dup)"=w245:string)  [unwired: 8 in]
        n100 = case shown="True" w241 {
          tunnel: w245 -> [_ w249]
          tunnel: [_ w248] -> w242
          frame False {
          }
          frame True {
            n101 = call "uuid.vi"() -> ("UUID"=w250:string)  [unwired: 11 in]
            n102 = call "Build Synchronous Message with Arguments.vi"("State With Arguments"="Message With Error", "Arguments (\"\")"=w250, "Target Module (\"\")"=w249) -> ("CSM Message String"=w248:string)  [unwired: 12 in]
          }
        }
        n103 = call <vilib>:"Add State(s) to Queue__JKI_lib_State_Machine.vi"("State(s) in Front (\"\")"=w242, "State(s) in (\"\")"=w243) -> ("States Out"=w244:string)  [unwired: 13 in]
      }
      frame "API: Test SyncMessage via API" {
        n104 = call "CSM - Check If Module Exists.vi"("CSM Name"=w271) -> ("error out"=w266:errorcluster, "Exist?"=w267:bool, "CSM Name (Dup)"=w270:string)  [unwired: 8 in]
        n105 = case shown="True" w267 {
          tunnel: w270 -> [_ w279]
          tunnel: [_ w278] -> w254
          tunnel: w256 -> [_ w277]
          tunnel: [_ w276] -> w263
          tunnel: [_ w275] -> w253
          tunnel: [_ w274] -> w259
          tunnel: [_ w273] -> w262
          frame False {
          }
          frame True {
            w276 = "Message" ("State With Arguments")
            n106 = call "uuid.vi"() -> ("UUID"=w274:string)  [unwired: 11 in]
            n107 = call "CSM - Wait and Send Message for Reply.vi"("State"=w276, "Current Module (\"\" to Generate an ID)"=w277, "Arguments (\"\")"=w274, "Target Module"=w279) -> ("Response"=w273:string, "Source CSM"=w275:string, "error out"=w278:errorcluster)  [unwired: 8 in, 1 out]
          }
        }
        n108 = call "CSM - Resolve Node Module.vi"("Node Name"=w256) -> ("CSM Module Name"=w255:string)  [unwired: 10 in]
        n109 = call "CSM - Resolve Node Module.vi"("Node Name"=w253) -> ("CSM Module Name"=w252:string)  [unwired: 10 in]
        n110 = Bundle By Name(cluster=T1 {"Arguments"="", "Response"="", "error"={"status"=FALSE, "code"=0, "source"=""}}, "Arguments"=w259, "Response"=w262, "error"=w254) -> (w257:T1)
        n111 = Concatenate Strings(w252, ":" ("string"), w263) -> (w261:string)
        n112 = call "CSM - Set Module Attribute.vi"("CSM Name"=w255, "Attribute"=w261, "Value"=w257) -> ("error out"=w260:errorcluster)  [unwired: 9 in, 3 out]
        n113 = call <vilib>:"Add State(s) to Queue__JKI_lib_State_Machine.vi"("State(s) in (\"\")"=w268) -> ("States Out"=w269:string)  [unwired: 14 in]
        n114 = Merge Errors(w260, w254, w266) -> (w265:errorcluster)
      }
      frame "API: Test SyncMessage With Error via API" {
        n115 = call "CSM - Check If Module Exists.vi"("CSM Name"=w299) -> ("error out"=w294:errorcluster, "Exist?"=w295:bool, "CSM Name (Dup)"=w298:string)  [unwired: 8 in]
        n116 = case shown="True" w295 {
          tunnel: w298 -> [_ w307]
          tunnel: [_ w306] -> w282
          tunnel: w284 -> [_ w305]
          tunnel: [_ w304] -> w291
          tunnel: [_ w303] -> w281
          tunnel: [_ w302] -> w287
          tunnel: [_ w301] -> w290
          frame False {
          }
          frame True {
            w304 = "Message With Error" ("State With Arguments")
            n117 = call "uuid.vi"() -> ("UUID"=w302:string)  [unwired: 11 in]
            n118 = call "CSM - Wait and Send Message for Reply.vi"("State"=w304, "Current Module (\"\" to Generate an ID)"=w305, "Arguments (\"\")"=w302, "Target Module"=w307) -> ("Response"=w301:string, "Source CSM"=w303:string, "error out"=w306:errorcluster)  [unwired: 8 in, 1 out]
          }
        }
        n119 = call "CSM - Resolve Node Module.vi"("Node Name"=w281) -> ("CSM Module Name"=w280:string)  [unwired: 10 in]
        n120 = Bundle By Name(cluster=T1 {"Arguments"="", "Response"="", "error"={"status"=FALSE, "code"=0, "source"=""}}, "Arguments"=w287, "Response"=w290, "error"=w282) -> (w286:T1)
        n121 = call "CSM - Resolve Node Module.vi"("Node Name"=w284) -> ("CSM Module Name"=w283:string)  [unwired: 10 in]
        n122 = Concatenate Strings(w280, ":" ("string"), w291) -> (w289:string)
        n123 = call "CSM - Set Module Attribute.vi"("CSM Name"=w283, "Attribute"=w289, "Value"=w286) -> ("error out"=w288:errorcluster)  [unwired: 9 in, 3 out]
        n124 = call <vilib>:"Add State(s) to Queue__JKI_lib_State_Machine.vi"("State(s) in (\"\")"=w296) -> ("States Out"=w297:string)  [unwired: 14 in]
        n125 = Merge Errors(w288, w282, w294) -> (w293:errorcluster)
      }
      frame "API: Test AsyncMessageWithReply" {
        n126 = call "CSM - Check If Module Exists.vi"("CSM Name"=w314) -> ("error out"=w308:errorcluster, "Exist?"=w309:bool, "CSM Name (Dup)"=w313:string)  [unwired: 8 in]
        n127 = case shown="True" w309 {
          tunnel: w313 -> [_ w317]
          tunnel: [_ w316] -> w310
          frame False {
          }
          frame True {
            n128 = call "uuid.vi"() -> ("UUID"=w318:string)  [unwired: 11 in]
            n129 = call-poly "Build Message with Arguments++.vi"("State With Arguments"="Message", "Arguments (\"\")"=w318, "Target Module (\"\")"=w317) -> ("CSM Message String"=w316:string)  [unwired: 12 in]
          }
        }
        n130 = call <vilib>:"Add State(s) to Queue__JKI_lib_State_Machine.vi"("State(s) in Front (\"\")"=w310, "State(s) in (\"\")"=w311) -> ("States Out"=w312:string)  [unwired: 13 in]
      }
      frame "API: Test AsyncMessageWithReply With Error" {
        n131 = call "CSM - Check If Module Exists.vi"("CSM Name"=w326) -> ("error out"=w320:errorcluster, "Exist?"=w321:bool, "CSM Name (Dup)"=w325:string)  [unwired: 8 in]
        n132 = case shown="True" w321 {
          tunnel: w325 -> [_ w330]
          tunnel: [_ w328] -> w322
          frame False {
          }
          frame True {
            n133 = call "uuid.vi"() -> ("UUID"=w329:string)  [unwired: 11 in]
            n134 = call-poly "Build Message with Arguments++.vi"("State With Arguments"="Message With Error", "Arguments (\"\")"=w329, "Target Module (\"\")"=w330) -> ("CSM Message String"=w328:string)  [unwired: 12 in]
          }
        }
        n135 = call <vilib>:"Add State(s) to Queue__JKI_lib_State_Machine.vi"("State(s) in Front (\"\")"=w322, "State(s) in (\"\")"=w323) -> ("States Out"=w324:string)  [unwired: 13 in]
      }
      frame "API: Test AsyncMessageWithoutReply" {
        n136 = call "CSM - Check If Module Exists.vi"("CSM Name"=w338) -> ("error out"=w332:errorcluster, "Exist?"=w333:bool, "CSM Name (Dup)"=w337:string)  [unwired: 8 in]
        n137 = case shown="True" w333 {
          tunnel: w337 -> [_ w343]
          tunnel: [_ w341] -> w334
          frame False {
          }
          frame True {
            n138 = call-poly "Build Message with Arguments++.vi"("State With Arguments"="AsyncMessageWithoutReply", "Arguments (\"\")"="123456789" ("Arguments (\"\")"), "Target Module (\"\")"=w343) -> ("CSM Message String"=w341:string)  [unwired: 12 in]
          }
        }
        n139 = call <vilib>:"Add State(s) to Queue__JKI_lib_State_Machine.vi"("State(s) in Front (\"\")"=w334, "State(s) in (\"\")"=w335) -> ("States Out"=w336:string)  [unwired: 13 in]
      }
      frame "API: Test AsyncMessageWithoutReply via API" {
        n140 = call "CSM - Check If Module Exists.vi"("CSM Name"=w352) -> ("error out"=w347:errorcluster, "Exist?"=w348:bool, "CSM Name (Dup)"=w351:string)  [unwired: 8 in]
        n141 = case shown="True" w348 {
          tunnel: w351 -> [_ w355]
          tunnel: w346 -> [_ w358]
          tunnel: [_ w354] -> w344
          frame False {
          }
          frame True {
            n142 = call "CSM - Wait and Post Message.vi"("State"="AsyncMessageWithoutReply" ("State With Arguments"), "Current Module (\"\" to Generate an ID)"=w358, "Arguments (\"\")"="123456789" ("Arguments (\"\")"), "Target Module"=w355) -> ("error out"=w354:errorcluster)  [unwired: 10 in, 1 out]
          }
        }
        n143 = call <vilib>:"Add State(s) to Queue__JKI_lib_State_Machine.vi"("State(s) in (\"\")"=w349) -> ("States Out"=w350:string)  [unwired: 14 in]
        n144 = Merge Errors(w344, w347) -> (w345:errorcluster)
      }
      frame "API: Test Argument" {
        n145 = call "uuid.vi"() -> ("UUID"=w364:string)  [unwired: 11 in]
        n146 = call "CSM - Convert HexStr to Data.vi"("HEX String"=w368) -> ("Variant"=w366:variant, "error out"=w367:errorcluster)  [unwired: 7 in]
        n147 = Bundle("", "UUID"=w364) -> (w362:cluster{string, "UUID":string})  [unwired: 1 in]
        n148 = Variant To Data(error in=w367, type=w362, Variant=w366) -> (data=w361:cluster{string, "UUID":string}, error out=w365:errorcluster)
        n149 = Unbundle(w361) -> (w360:string, "UUID"=w359:string)
        n150 = call "CSM - Check If Module Exists.vi"("Error In"=w365, "CSM Name"=w360) -> ("error out"=w369:errorcluster, "Exist?"=w370:bool, "CSM Name (Dup)"=w374:string)  [unwired: 7 in]
        n151 = case shown="True" w370 {
          tunnel: w374 -> [_ w378]
          tunnel: [_ w377] -> w371
          tunnel: w359 -> [_ w376]
          frame False {
          }
          frame True {
            n152 = call "Build Synchronous Message with Arguments.vi"("State With Arguments"="ArgumentTest", "Arguments (\"\")"=w376, "Target Module (\"\")"=w378) -> ("CSM Message String"=w377:string)  [unwired: 12 in]
          }
        }
        n153 = call <vilib>:"Add State(s) to Queue__JKI_lib_State_Machine.vi"("State(s) in Front (\"\")"=w371, "State(s) in (\"\")"=w372) -> ("States Out"=w373:string)  [unwired: 13 in]
      }
      frame "API: Test Response With Error" {
        n154 = call "CSM - Check If Module Exists.vi"("CSM Name"=w386) -> ("error out"=w380:errorcluster, "Exist?"=w381:bool, "CSM Name (Dup)"=w385:string)  [unwired: 8 in]
        n155 = case shown="True" w381 {
          tunnel: w385 -> [_ w389]
          tunnel: [_ w388] -> w382
          frame False {
          }
          frame True {
            n156 = call "uuid.vi"() -> ("UUID"=w390:string)  [unwired: 11 in]
            n157 = call "Build Synchronous Message with Arguments.vi"("State With Arguments"="Response With Error", "Arguments (\"\")"=w390, "Target Module (\"\")"=w389) -> ("CSM Message String"=w388:string)  [unwired: 12 in]
          }
        }
        n158 = call <vilib>:"Add State(s) to Queue__JKI_lib_State_Machine.vi"("State(s) in Front (\"\")"=w382, "State(s) in (\"\")"=w383) -> ("States Out"=w384:string)  [unwired: 13 in]
      }
      frame "API: Test MacroWithSubMessages" {
        n159 = call <vilib>:"Build State String with Arguments__JKI_lib_State_Machine.vi"("Arguments (\"\")"=w393, "State"="Macro: Test MacroWithSubMessages") -> ("State with Arguments"=w392:string)  [unwired: 4 in]
        n160 = call <vilib>:"Add State(s) to Queue__JKI_lib_State_Machine.vi"("State(s) in Front (\"\")"=w392, "State(s) in (\"\")"=w396) -> ("States Out"=w395:string)  [unwired: 13 in]
      }
      frame "API: Test MacroWithSubAndPostMessages" {
        n161 = call <vilib>:"Build State String with Arguments__JKI_lib_State_Machine.vi"("Arguments (\"\")"=w400, "State"="Macro: Test MacroWithSubAndPostMessages") -> ("State with Arguments"=w399:string)  [unwired: 4 in]
        n162 = call <vilib>:"Add State(s) to Queue__JKI_lib_State_Machine.vi"("State(s) in Front (\"\")"=w399, "State(s) in (\"\")"=w403) -> ("States Out"=w402:string)  [unwired: 13 in]
      }
      frame "API: Test MacroWithNonLocalSubMessages" {
        n163 = call <vilib>:"Build State String with Arguments__JKI_lib_State_Machine.vi"("Arguments (\"\")"=w407, "State"="Macro: TestMacroWithNonLocalSubMessages") -> ("State with Arguments"=w406:string)  [unwired: 4 in]
        n164 = call <vilib>:"Add State(s) to Queue__JKI_lib_State_Machine.vi"("State(s) in Front (\"\")"=w406, "State(s) in (\"\")"=w410) -> ("States Out"=w409:string)  [unwired: 13 in]
      }
      frame "API: Test Register State" {
        n165 = call <vilib>:"Build State String with Arguments__JKI_lib_State_Machine.vi"("Arguments (\"\")"=w414, "State"="Test Status") -> ("State with Arguments"=w413:string)  [unwired: 4 in]
        n166 = call <vilib>:"Add State(s) to Queue__JKI_lib_State_Machine.vi"("State(s) in Front (\"\")"=w413, "State(s) in (\"\")"=w417) -> ("States Out"=w416:string)  [unwired: 13 in]
      }
      frame "API: Test Register State Argument Info" {
        n167 = call <vilib>:"Build State String with Arguments__JKI_lib_State_Machine.vi"("Arguments (\"\")"=w421, "State"="Register State Argument Info") -> ("State with Arguments"=w420:string)  [unwired: 4 in]
        n168 = call <vilib>:"Add State(s) to Queue__JKI_lib_State_Machine.vi"("State(s) in Front (\"\")"=w420, "State(s) in (\"\")"=w424) -> ("States Out"=w423:string)  [unwired: 13 in]
      }
      frame "API: Test Register Status" {
        n169 = call <vilib>:"Build State String with Arguments__JKI_lib_State_Machine.vi"("Arguments (\"\")"=w428, "State"="Register Status") -> ("State with Arguments"=w427:string)  [unwired: 4 in]
        n170 = call <vilib>:"Add State(s) to Queue__JKI_lib_State_Machine.vi"("State(s) in Front (\"\")"=w427, "State(s) in (\"\")"=w431) -> ("States Out"=w430:string)  [unwired: 13 in]
      }
      frame "API: Test Register Interrupt" {
        n171 = call <vilib>:"Build State String with Arguments__JKI_lib_State_Machine.vi"("Arguments (\"\")"=w435, "State"="Register Interrupt") -> ("State with Arguments"=w434:string)  [unwired: 4 in]
        n172 = call <vilib>:"Add State(s) to Queue__JKI_lib_State_Machine.vi"("State(s) in Front (\"\")"=w434, "State(s) in (\"\")"=w438) -> ("States Out"=w437:string)  [unwired: 13 in]
      }
      frame "API: Test Register Status Argument Info" {
        n173 = call <vilib>:"Build State String with Arguments__JKI_lib_State_Machine.vi"("Arguments (\"\")"=w442, "State"="Register Status Argument Info") -> ("State with Arguments"=w441:string)  [unwired: 4 in]
        n174 = call <vilib>:"Add State(s) to Queue__JKI_lib_State_Machine.vi"("State(s) in Front (\"\")"=w441, "State(s) in (\"\")"=w445) -> ("States Out"=w444:string)  [unwired: 13 in]
      }
      frame "API: Test Status A" {
        n175 = call <vilib>:"Build State String with Arguments__JKI_lib_State_Machine.vi"("Arguments (\"\")"=w449, "State"="Broadcast Status A") -> ("State with Arguments"=w450:string)  [unwired: 4 in]
        n176 = call <vilib>:"Add State(s) to Queue__JKI_lib_State_Machine.vi"("State(s) in Front (\"\")"=w450, "State(s) in (\"\")"=w452) -> ("States Out"=w451:string)  [unwired: 13 in]
      }
      frame "API: Test State A" {
        n177 = call <vilib>:"Build State String with Arguments__JKI_lib_State_Machine.vi"("Arguments (\"\")"=w456, "State"="State A") -> ("State with Arguments"=w457:string)  [unwired: 4 in]
        n178 = call <vilib>:"Add State(s) to Queue__JKI_lib_State_Machine.vi"("State(s) in Front (\"\")"=w457, "State(s) in (\"\")"=w459) -> ("States Out"=w458:string)  [unwired: 13 in]
      }
      frame "API: Test State B" {
        n179 = call <vilib>:"Build State String with Arguments__JKI_lib_State_Machine.vi"("Arguments (\"\")"=w463, "State"="State B") -> ("State with Arguments"=w464:string)  [unwired: 4 in]
        n180 = call <vilib>:"Add State(s) to Queue__JKI_lib_State_Machine.vi"("State(s) in Front (\"\")"=w464, "State(s) in (\"\")"=w466) -> ("States Out"=w465:string)  [unwired: 13 in]
      }
      frame "API: Test Status B" {
        n181 = call <vilib>:"Build State String with Arguments__JKI_lib_State_Machine.vi"("Arguments (\"\")"=w470, "State"="Broadcast Status B") -> ("State with Arguments"=w471:string)  [unwired: 4 in]
        n182 = call <vilib>:"Add State(s) to Queue__JKI_lib_State_Machine.vi"("State(s) in Front (\"\")"=w471, "State(s) in (\"\")"=w473) -> ("States Out"=w472:string)  [unwired: 13 in]
      }
      frame "API: Local Registration" {
        # "Test Status @ From >> Handler Message @ To -><register>"
        n183 = call "CSM - Resolve Node Module.vi"("Node Name"=w480) -> ("CSM Module Name"=w476:string)  [unwired: 10 in]
        n184 = call-poly "Build Message with Arguments++.vi"("Target CSM"=w477, "Source CSM (* as Default)"=w476, "Status"="Test Status", "API (If \"\", Same As \"Status\")"="Handler Message") -> ("CSM Message String"=w478:string)  [unwired: 11 in]
        n185 = call <vilib>:"Add State(s) to Queue__JKI_lib_State_Machine.vi"("State(s) in Front (\"\")"=w478, "State(s) in (\"\")"=w484) -> ("States Out"=w483:string)  [unwired: 13 in]
      }
      frame "API: Local Registration II" {
        # "Test Status @ From >> Handler Message -><register>"
        n186 = call "CSM - Resolve Node Module.vi"("Node Name"=w488) -> ("CSM Module Name"=w485:string)  [unwired: 10 in]
        n187 = call-poly "Build Message with Arguments++.vi"("Source CSM (* as Default)"=w485, "Status"="Test Status", "API (If \"\", Same As \"Status\")"="Handler Message") -> ("CSM Message String"=w486:string)  [unwired: 12 in]
        n188 = call <vilib>:"Add State(s) to Queue__JKI_lib_State_Machine.vi"("State(s) in Front (\"\")"=w486, "State(s) in (\"\")"=w492) -> ("States Out"=w491:string)  [unwired: 13 in]
      }
      frame "API: Local Unregistration" {
        # "Test Status @ From >> Handler Message @ To -><unregister>"
        n189 = call "CSM - Resolve Node Module.vi"("Node Name"=w497) -> ("CSM Module Name"=w493:string)  [unwired: 10 in]
        n190 = call-poly "Build Message with Arguments++.vi"("Target CSM"=w494, "Source CSM (* as Default)"=w493, "Status"="Test Status", "API (If \"\", Same As \"Status\")"="Handler Message") -> ("CSM Message String"=w495:string)  [unwired: 11 in]
        n191 = call <vilib>:"Add State(s) to Queue__JKI_lib_State_Machine.vi"("State(s) in Front (\"\")"=w495, "State(s) in (\"\")"=w501) -> ("States Out"=w500:string)  [unwired: 13 in]
      }
      frame "API: Local Registration via API" {
        # "Test Status @ From >> Handler Message @ To -><register>"
        n192 = call "CSM - Resolve Node Module.vi"("Node Name"=w507) -> ("CSM Module Name"=w503:string)  [unwired: 10 in]
        n193 = call "CSM - Register Broadcast.vi"("CSM Name(Empty for Broadcast Event)"=w502, "Source CSM Name (* as Default)"=w503, "Trigger"="Test Status", "API (If \"\", Same as Trigger)"="Handler Message") -> ("error out"=w506:errorcluster)  [unwired: 10 in, 1 out]
        n194 = call <vilib>:"Add State(s) to Queue__JKI_lib_State_Machine.vi"("State(s) in (\"\")"=w510) -> ("States Out"=w509:string)  [unwired: 14 in]
      }
      frame "API: Local Unregistration via API" {
        # "Test Status @ From >> Handler Message @ To -><unregister>"
        n195 = call "CSM - Resolve Node Module.vi"("Node Name"=w516) -> ("CSM Module Name"=w512:string)  [unwired: 10 in]
        n196 = call "CSM - Unregister Broadcast.vi"("CSM Name(Empty for Broadcast Event)"=w511, "Source CSM Name (* as Default)"=w512, "Trigger"="Test Status", "API (\"*\" as Default)"="Handler Message") -> ("error out"=w515:errorcluster)  [unwired: 10 in, 1 out]
        n197 = call <vilib>:"Add State(s) to Queue__JKI_lib_State_Machine.vi"("State(s) in (\"\")"=w519) -> ("States Out"=w518:string)  [unwired: 14 in]
      }
      frame "API: Start CSM Loop" {
        n198 = call <vilib>:"Add State(s) to Queue__JKI_lib_State_Machine.vi"("State(s) in Front (\"\")"="Macro: Start CSM Loop" ("State(s) in Front (\"\")"), "State(s) in (\"\")"=w522) -> ("States Out"=w521:string)  [unwired: 13 in]
      }
      frame "API: Stop CSM Loop" {
        n199 = call <vilib>:"Add State(s) to Queue__JKI_lib_State_Machine.vi"("State(s) in Front (\"\")"="Macro: Stop CSM Loop" ("State(s) in Front (\"\")"), "State(s) in (\"\")"=w526) -> ("States Out"=w525:string)  [unwired: 13 in]
      }
      frame "API: API2" {
        # "#CSM API Example\nCopy/Rename this case for your own API"
        # "unpack Hex String  to Variant\nif complex parameter is needed."
        n200 = call "CSM - Convert HexStr to Data.vi"("HEX String"=w531) -> ()  [unwired: 7 in, 2 out]
        n201 = disable-structure shown="Enabled" {
          disable-tunnel: [w534 "API2 Response"] -> w530
          frame Disabled {
            # "pack variant to hexstr \nif complex response is needed."
            # "complex Response"
            n202 = call "CSM - Convert Data to HexStr.vi"() -> ("HEX String (0-9,A-F)"=w534:string)  [unwired: 9 in]
          }
          frame Enabled {
          }
        }
      }
      frame "---------- Action ----------" {
        # "#CSM \"Category Seperator\"\nDo not put any code in this frame."
        n203 = call <vilib>:"Add State(s) to Queue__JKI_lib_State_Machine.vi"("State(s) in (\"\")"=w538) -> ("States Out"=w537:string)  [unwired: 14 in]
      }
      frame "Action: action1" {
        # "#CSM \"Internal State\"\nThis category is used for holding internal states"
        n204 = call <vilib>:"Add State(s) to Queue__JKI_lib_State_Machine.vi"("State(s) in (\"\")"=w541) -> ("States Out"=w540:string)  [unwired: 14 in]
      }
      frame "Start CSM Loop" {
        n205 = Bundle By Name(cluster=w544, "CSM Loop Counter"=0) -> (w543:T6)
      }
      frame "Run CSM Loop" {
        # "Set loop rate to 1ms"
        n206 = Wait (ms)(milliseconds to wait=u32 1) -> ()  [unwired: 1 out]
        n207 = Unbundle By Name(w555) -> ("CSM Loop Counter"=w554:i32)
        n208 = call "CSM - Resolve Node Module.vi"("Node Name"=w551) -> ("CSM Module Name"=w550:string)  [unwired: 10 in]
        n209 = Increment(x=w554) -> (x+1=w548:i32)
        n210 = Bundle By Name(cluster=w555, "CSM Loop Counter"=w548) -> (w553:T6)
        n211 = call "CSM - Set Module Attribute.vi"("CSM Name"=w550, "Attribute"=w549, "Value"=w548) -> ("error out"=w547:errorcluster)  [unwired: 9 in, 3 out]
        n212 = call "CSMLS - Append Continuous State.vi"("Append? (T)"=TRUE, "Continous State"=w549, "States Queue"=w557) -> ("Remaining States"=w558:string)  [unwired: 8 in]
      }
      frame "Stop CSM Loop" {
        w560 = -1 ("CSM Loop Counter")
        n213 = call "CSM - Resolve Node Module.vi"("Node Name"=w561) -> ("CSM Module Name"=w563:string)  [unwired: 10 in]
        n214 = Bundle By Name(cluster=w565, "CSM Loop Counter"=w560) -> (w564:T6)
        n215 = call "CSM - Set Module Attribute.vi"("CSM Name"=w563, "Attribute"=w559, "Value"=w560) -> ("error out"=w562:errorcluster)  [unwired: 9 in, 3 out]
        n216 = call "CSMLS - Remove Loop Tag and previous State(s) to Break.vi"("States Queue"=w567) -> ("Remaining States"=w566:string)  [unwired: 10 in]
        n217 = call <vilib>:"Add State(s) to Queue__JKI_lib_State_Machine.vi"("State(s) in (\"\")"=w566) -> ("States Out"=w568:string)  [unwired: 14 in]
      }
      frame "Test Status" {
        n218 = call <vilib>:"Add State(s) to Queue__JKI_lib_State_Machine.vi"("State(s) in (\"\")"=w572) -> ("States Out"=w571:string)  [unwired: 14 in]
      }
      frame "Register State Argument Info" {
        n219 = call "CSM - Resolve Node Module.vi"("Node Name"=w575) -> ("CSM Module Name"=w576:string)  [unwired: 10 in]
        n220 = Concatenate Strings(w573, "+", w576) -> (w574:string)
        n221 = call <vilib>:"Add State(s) to Queue__JKI_lib_State_Machine.vi"("State(s) in (\"\")"=w578) -> ("States Out"=w580:string)  [unwired: 14 in]
      }
      frame "Register Status" {
        n222 = call <vilib>:"Build State String with Arguments__JKI_lib_State_Machine.vi"("Arguments (\"\")"=w581, "State"="Test Status") -> ("State with Arguments"=w583:string)  [unwired: 4 in]
        n223 = call "CSM - Broadcast Status Change.vi"("Status With Arguments"=w583, "State Queue"=w585) -> ("Remaining States"=w582:string)  [unwired: 13 in]
      }
      frame "Register Interrupt" {
        n224 = call-poly "Build Message with Arguments++.vi"("State With Arguments"="Test Interrupt", "Arguments (\"\")"=w590) -> ("CSM Message String"=w589:string)  [unwired: 13 in]
        n225 = call <vilib>:"Add State(s) to Queue__JKI_lib_State_Machine.vi"("State(s) in Front (\"\")"=w589, "State(s) in (\"\")"=w588) -> ("States Out"=w587:string)  [unwired: 13 in]
      }
      frame "Register Status Argument Info" {
        w597 = "Test Status Argument Info"
        n226 = call "CSM - Resolve Node Module.vi"("Node Name"=w595) -> ("CSM Module Name"=w594:string)  [unwired: 10 in]
        n227 = Concatenate Strings(w597, "+", w594) -> (w593:string)
        n228 = call <vilib>:"Build State String with Arguments__JKI_lib_State_Machine.vi"("Arguments (\"\")"=w593, "State"=w597) -> ("State with Arguments"=w599:string)  [unwired: 4 in]
        n229 = call "CSM - Broadcast Status Change.vi"("Status With Arguments"=w599, "State Queue"=w600) -> ("Remaining States"=w598:string)  [unwired: 13 in]
      }
      frame "Broadcast Status A" {
        n230 = call <vilib>:"Build State String with Arguments__JKI_lib_State_Machine.vi"("Arguments (\"\")"=w602, "State"="Status A") -> ("State with Arguments"=w604:string)  [unwired: 4 in]
        n231 = call "CSM - Broadcast Status Change.vi"("Status With Arguments"=w604, "State Queue"=w606) -> ("Remaining States"=w603:string)  [unwired: 13 in]
      }
      frame "Broadcast Status B" {
        n232 = call <vilib>:"Build State String with Arguments__JKI_lib_State_Machine.vi"("Arguments (\"\")"=w608, "State"="Status B") -> ("State with Arguments"=w610:string)  [unwired: 4 in]
        n233 = call "CSM - Broadcast Status Change.vi"("Status With Arguments"=w610, "State Queue"=w612) -> ("Remaining States"=w609:string)  [unwired: 13 in]
      }
      frame "State A" {
        n234 = call <vilib>:"Add State(s) to Queue__JKI_lib_State_Machine.vi"("State(s) in (\"\")"=w616) -> ("States Out"=w615:string)  [unwired: 14 in]
      }
      frame "State B" {
        n235 = call <vilib>:"Add State(s) to Queue__JKI_lib_State_Machine.vi"("State(s) in (\"\")"=w621) -> ("States Out"=w620:string)  [unwired: 14 in]
      }
      frame "Message" {
      }
      frame "SubMessage1" {
      }
      frame "SubMessage2" {
      }
      frame "SubMessage3" {
        n236 = call "CSM - Resolve Node Module.vi"("Node Name"=w641) -> ("CSM Module Name"=w640:string)  [unwired: 10 in]
        n237 = call "CSM - Set Module Attribute.vi"("CSM Name"=w640, "Attribute"=w639, "Value"=w638) -> ("error out"=w636:errorcluster)  [unwired: 9 in, 3 out]
        n238 = Merge Errors(w636, w644) -> (w637:errorcluster)
      }
      frame "PostMessage1" {
      }
      frame "Message With Error" {
        n239 = Merge Errors(errorcluster {"status"=TRUE, "code"=1234567898, "source"="Simulated Error\nwill be sent to Response case"} ("error out"), w650) -> (w649:errorcluster)
      }
      frame "Response With Error" {
        n240 = Merge Errors(errorcluster {"status"=TRUE, "code"=1234567898, "source"="Simulated Error"} ("error out"), w656) -> (w655:errorcluster)
      }
      frame "ArgumentTest" {
        n241 = call "CSM - Resolve Node Module.vi"("Node Name"=w666) -> ("CSM Module Name"=w665:string)  [unwired: 10 in]
        n242 = call "CSM - Set Module Attribute.vi"("CSM Name"=w665, "Attribute"=w663, "Value"=w664) -> ("error out"=w661:errorcluster)  [unwired: 9 in, 3 out]
        n243 = Merge Errors(w661, w669) -> (w662:errorcluster)
      }
      frame "AsyncMessageWithoutReply" {
        # "123456789 string constant"
        n244 = call "CSM - Resolve Node Module.vi"("Node Name"=w673) -> ("CSM Module Name"=w672:string)  [unwired: 10 in]
        n245 = call "CSM - Set Module Attribute.vi"("CSM Name"=w672, "Attribute"=w674, "Value"=w675) -> ("error out"=w670:errorcluster)  [unwired: 9 in, 3 out]
        n246 = Merge Errors(w670, w678) -> (w671:errorcluster)
      }
      frame "Handler Message" {
        n247 = call "CSM - Resolve Node Module.vi"("Node Name"=w684) -> ("CSM Module Name"=w683:string)  [unwired: 10 in]
        n248 = call "CSM - Set Module Attribute.vi"("CSM Name"=w683, "Attribute"=w681, "Value"=w680) -> ("error out"=w679:errorcluster)  [unwired: 9 in, 3 out]
        n249 = Merge Errors(w687, w679) -> (w682:errorcluster)
      }
      frame "Handler Message With Counter" {
        n250 = Unbundle By Name(w693) -> ("Counter"=w694:u32)
        n251 = Decimal String To Number(string=w691) -> (number=w688:i32)  [unwired: 2 in, 1 out]
        n252 = Increment(x=w694) -> (x+1=w689:u32)
        n253 = Bundle By Name(cluster=w693, "Counter"=w689) -> (w692:T6)
        n254 = Equal?(x=w689, y=w688) -> (x = y?=w690:bool)
        n255 = call "CSM - Resolve Node Module.vi"("Node Name"=w699) -> ("CSM Module Name"=w698:string)  [unwired: 10 in]
        n256 = case shown="True" w690 {
          tunnel: w698 -> [_ w705]
          tunnel: w696 -> [_ w704]
          tunnel: [_ w703] -> w695
          tunnel: w689 -> [_ w702]
          frame False {
          }
          frame True {
            n257 = call "CSM - Set Module Attribute.vi"("CSM Name"=w705, "Attribute"=w704, "Value"=w702) -> ("error out"=w703:errorcluster)  [unwired: 9 in, 3 out]
          }
        }
        n258 = Merge Errors(w701, w695) -> (w697:errorcluster)
      }
      frame "Reset Counter" {
        # "#CSM \"Internal State\"\nThis category is used for holding internal states"
        n259 = Bundle By Name(cluster=w708, "Counter"=u32 0) -> (w706:T6)
        n260 = call <vilib>:"Add State(s) to Queue__JKI_lib_State_Machine.vi"("State(s) in (\"\")"=w710) -> ("States Out"=w709:string)  [unwired: 14 in]
      }
    }
  }
